vi "get_image_sequences.vi"(8 "Error In":errorcluster, 10 "Sample":string, 11 "File Path":path) -> (0 "Error Out":errorcluster, 1 "File Paths":path[][](array[path]), 2 "Phiin":dbl[](array[numeric]), 3 "Xi":dbl[](array[numeric]), 5 "Image Names":string[][](array[string]))   [LabVIEW 2019]
doc: "Gets image sequences (pairs of xi and phiin angles)"
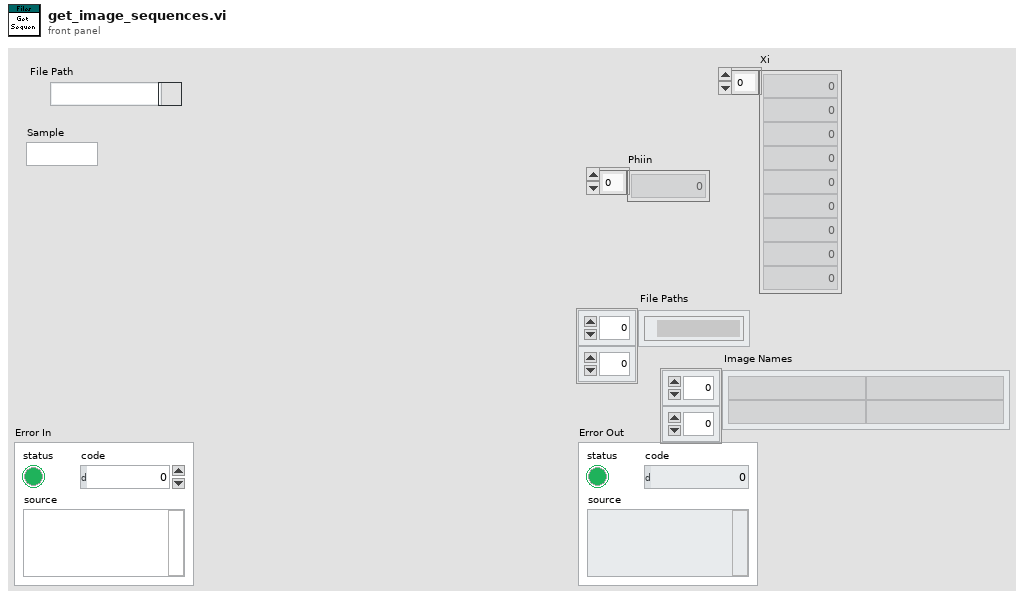
[diagram p1: front panel]
types:
  T1 = typedef "image_property_cluster_typedef.ctl" = cluster{"Stage Angle":dbl, "Sample Angle":dbl, "Polarizer 1 Angle":dbl, "Polarizer 2 Angle":dbl, "Sample Name":string}
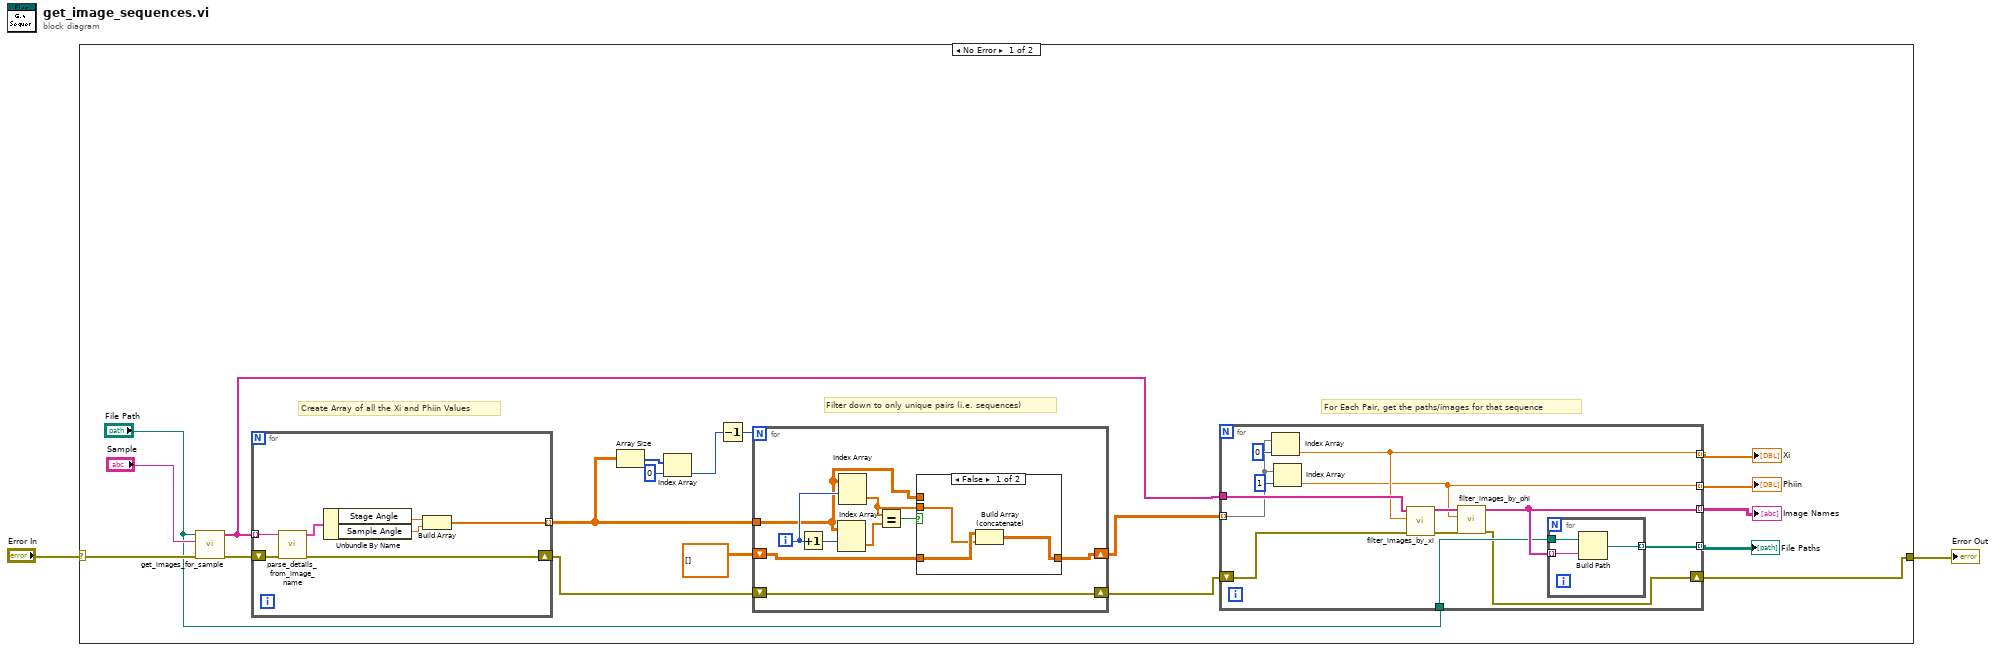
[diagram p0: block diagram]
diagram:
  n1 = case shown="No Error" "Error In" {
    selector: "Error In" -> [w20 w58]
    tunnel: [w3 w58] -> w1
    frame No Error {
      # "For Each Pair, get the paths/images for that sequence"
      # "Filter down to only unique pairs (i.e. sequences)"
      # "Create Array of all the Xi and Phiin Values"
      n2 = call "get_images_for_sample.vi"("Error In"=w20, "Sample"="Sample", "File Path"="File Path") -> ("Error Out"=w19:errorcluster, "Image Names"=w11:string[])  [unwired: 7 in]
      n3 = for {
        tunnel: w11 -> [w56] mode=indexing
        shift-right: [w54] -> w10
        shift-left: w19 -> [w57]
        tunnel: [w51] -> w14 mode=indexing
        n4 = call "parse_details_from_image_name.vi"("Error In"=w57, "Image Name"=w56) -> ("Error Out"=w54:errorcluster, "Image Properties"=w55:T1)  [unwired: 8 in]
        n5 = Unbundle By Name(w55) -> ("Stage Angle"=w53:dbl, "Sample Angle"=w52:dbl)
        n6 = Build Array(w53, w52) -> (w51:dbl[])
      }
      n7 = Array Size(array=w14) -> (size(s)=w18:i32[])
      n8 = Index Array(array=w18, index=0) -> (element=w15:i32)
      n9 = Decrement(x=w15) -> (x-1=w16:i32)
      n10 = for {
        N: w16 -> [_]
        tunnel: w14 -> [w42]
        shift-right: [w41] -> w12
        shift-left: dbl[][] [] -> [w40]
        shift-right: [w38] -> w9
        shift-left: w10 -> [w38]
        i -> [w45]
        n11 = Increment(x=w45) -> (x+1=w46:i32)
        n12 = Index Array(array=w42, index (row)=w46) -> (element=w44:dbl[])  [unwired: 1 in]
        n13 = Index Array(array=w42, index (row)=w45) -> (element=w39:dbl[])  [unwired: 1 in]
        n14 = Equal?(x=w39, y=w44) -> (x = y?=w43:bool)
        n15 = case shown="False" w43 {
          tunnel: w42 -> [_ _]
          tunnel: [w47 w50] -> w41
          tunnel: w40 -> [w49 w50]
          tunnel: w39 -> [w48 _]
          frame False {
            n16 = Build Array (concatenate)(w49, w48) -> (w47:dbl[][])
          }
          frame True {
          }
        }
      }
      n17 = for {
        tunnel: w12 -> [w31] mode=indexing
        tunnel: w11 -> [w33]
        shift-right: [w22] -> w3
        shift-left: w9 -> [w34]
        tunnel: [w27] -> w4 mode=indexing
        tunnel: "File Path" -> [w26]
        tunnel: [w25] -> w5 mode=indexing
        tunnel: [w24] -> w6 mode=indexing
        tunnel: [w23] -> w7 mode=indexing
        n18 = Index Array(array=w31, index=0) -> (element=w24:dbl)
        n19 = Index Array(array=w31, index=1) -> (element=w23:dbl)
        n20 = call "filter_images_by_xi.vi"("Error In"=w34, "Xi"=w24, "Image Names"=w33) -> ("Error Out"=w28:errorcluster, "Filtered Image Names"=w29:string[])  [unwired: 7 in]
        n21 = call "filter_images_by_phi.vi"("Error In"=w28, "Phi"=w23, "Image Names"=w29) -> ("Error Out"=w22:errorcluster, "Filtered Image Names"=w27:string[])  [unwired: 7 in]
        n22 = for {
          tunnel: w27 -> [w37] mode=indexing
          tunnel: w26 -> [w36]
          tunnel: [w35] -> w25 mode=indexing
          n23 = Build Path(base path=w36, name or relative path=w37) -> (appended path=w35:path)
        }
      }
      "Phiin" <- w7
      "Xi" <- w6
      "File Paths" <- w5
      "Image Names" <- w4
    }
    frame Error {
    }
  }
  "Error Out" <- w1
